vi "G#Interface_AbstractMethod.vi"(0 "reference in":refnum<class "G#Interface.lvclass">, 5 "error in (no error)":errorcluster) -> (14 "reference out":refnum<class "G#Interface.lvclass">, 19 "error out":errorcluster)   [LabVIEW 2017, in "G#Interface.lvclass"]
doc: "Sets an error if this method is not overridden."
uses:
  <vilib>/addons/_AddQ/G#Interface/G#Interface.lvclass
  C:/Program Files (x86)/National Instruments/LabVIEW 2017/vi.lib/addons/_AddQ/G#Object/G#Object.lvclass
  <vilib>/addons/_AddQ/G#Interface/G#Interface.lvclass/G#Interface.ctl
  <vilib>/addons/_AddQ/G#Object/G#Object.lvclass
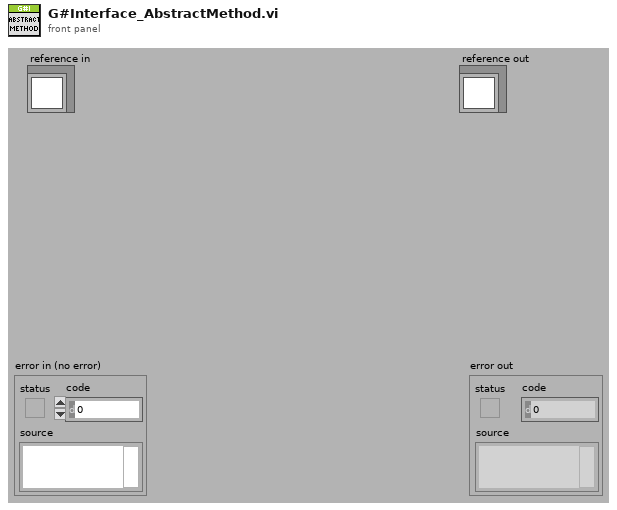
[diagram p1: front panel]
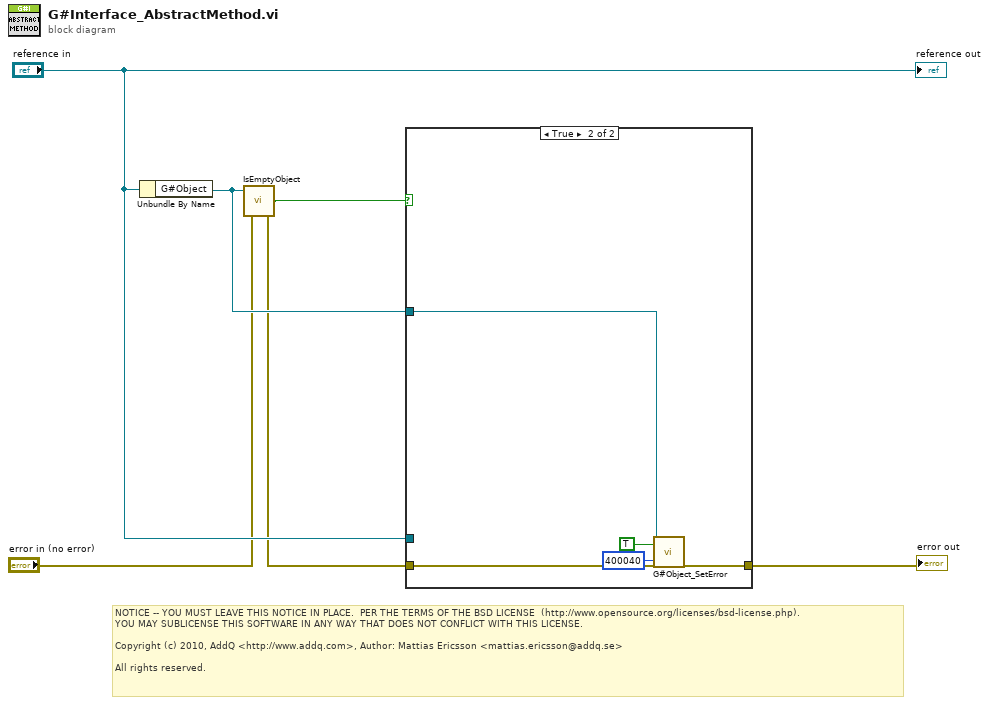
[diagram p0: block diagram]
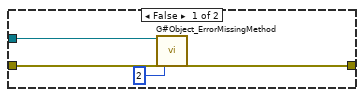
[diagram p2: hidden frame]
diagram:
  # "NOTICE -- YOU MUST LEAVE THIS NOTICE IN PLACE.  PER THE TERMS OF THE BSD LICENSE  (http://www.opensource.org/licenses/bsd-license.php).\nYOU MAY SUBLICENSE THIS SOFTWARE IN ANY WAY THAT DOES NOT CONFLICT WITH THIS LICENSE.\n\nCopyright (c) 2010, AddQ <http://www.addq.com>, Author: Mattias Ericsson <mattias.ericsson@addq.se>\n\nAll rights reserved."
  n1 = Unbundle By Name("reference in") -> ("G#Object"=w3:refnum<class "G#Object.lvclass">)
  n2 = call-dynamic "IsEmptyObject.vi"("error in (no error)"="error in (no error)", "reference in"=w3) -> ("error out"=w1:errorcluster, "is empty?"=w4:bool)  [unwired: 1 in, 1 out]
  n3 = case shown="True" w4 {
    tunnel: [w10 w15] -> w5
    tunnel: w1 -> [w9 w14]
    tunnel: "reference in" -> [w8 _]
    tunnel: w3 -> [_ w13]
    frame False {
      n4 = call <vilib>:"G#Object_ErrorMissingMethod.vi"("reference in"=w8, "error in (no error)"=w9, "call depth (1)"=2 ("CallerNo(1)")) -> ("error out"=w10:errorcluster)  [unwired: 15 in, 1 out]
    }
    frame True {
      n5 = call <vilib>:"G#Object_SetError.vi"("reference in"=w13, "error (F)"=TRUE ("error"), "code"=400040, "error in (no error)"=w14) -> ("error out"=w15:errorcluster)  [unwired: 15 in]
    }
  }
  "error out" <- w5
  "reference out" <- "reference in"
